vi "hidSPD Read Signal Board.vi"(8 "error in (no error)":errorcluster, 11 "spdDevSession in":T2={"spdRef"=0, "connected"=FALSE, "spdName"="", "specification"={"diod case"=enum."default", "type"=enum."Unknown", "frequency"=enum."Unknown"}, "hidSPD.Controller"={"TSet"=0.0, "HV_bias"=0.0, "DDS_stb_code"=0}, "hidSPD.Sturtup Values"={"TSet"=0.0, "HV_bias"=0.0, "DDS_stb_code"=0}} {"hidSPD.Sturtup Values"."HV_bias" format="%#_6p, V"; "hidSPD.Sturtup Values"."TSet" format="%#_6p, DegC"; "hidSPD.Controller"."HV_bias" format="%#_6p, V"; "hidSPD.Controller"."TSet" format="%#_6p, DegC"}) -> (0 "error out":errorcluster, 2 "Signal Board params":T1, 3 "spdDevSession out":T2={"spdRef"=0, "connected"=FALSE, "spdName"="", "specification"={"diod case"=enum."default", "type"=enum."Unknown", "frequency"=enum."Unknown"}, "hidSPD.Controller"={"TSet"=0.0, "HV_bias"=0.0, "DDS_stb_code"=0}, "hidSPD.Sturtup Values"={"TSet"=0.0, "HV_bias"=0.0, "DDS_stb_code"=0}} {"hidSPD.Sturtup Values"."HV_bias" format="%#_6p, V"; "hidSPD.Sturtup Values"."TSet" format="%#_6p, DegC"; "hidSPD.Controller"."HV_bias" format="%#_6p, V"; "hidSPD.Controller"."TSet" format="%#_6p, DegC"})   [LabVIEW 2018, in "hidSPDLibForLabView.lvlib"]
uses:
  hidSPDLibForLabView.lvlib
  hidSPD Controls/hidSPD Device Session.ctl
  hidSPD Controls/hidSPD.SPD specification.ctl
  hidSPD Controls/hidSPD SPD Diod Case.ctl
  hidSPD Controls/hidSPD SPD Type.ctl
  hidSPD Controls/hidSPD.STB Frequency.ctl
  hidSPD Controls/hidSPD Controller.ctl
  hidSPD Controls/hidSPD Controller Signal Report.ctl
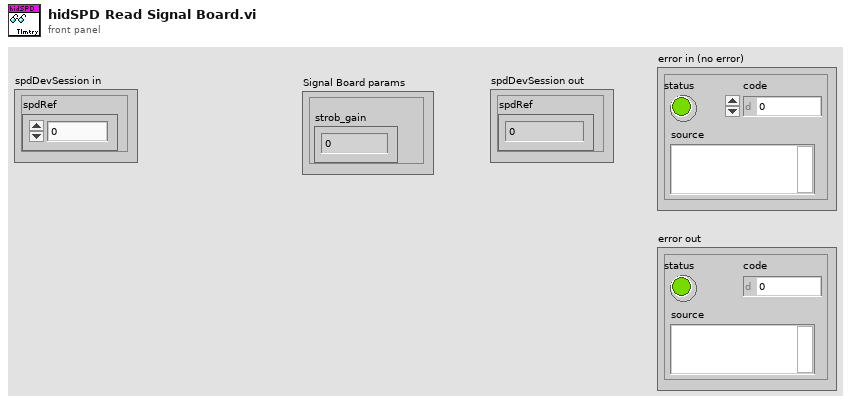
[diagram p1: front panel]
types:
  T1 = typedef "hidSPDLibForLabView.lvlib/hidSPD Controller Signal Report.ctl" = cluster{"strob_gain":i8, "receive_gain":i8, "positive_bias":i32, "negative_bias":i32, "deadtime":i16, "insensitivity":i16, "deadtime_strobe":i8, "dt_on":i8, "frequency":i16, "pllpwr":i8, "rvset":i16, "dvset":i16}
  T2 = typedef "hidSPDLibForLabView.lvlib/hidSPD Device Session.ctl" = cluster{"spdRef":u64, "connected":bool, "spdName":string, "specification":T3, "hidSPD.Controller":T7, "hidSPD.Sturtup Values":T7}
  T3 = typedef "hidSPDLibForLabView.lvlib/hidSPD.SPD specification.ctl" = cluster{"diod case":T4, "type":T5, "frequency":T6}
  T4 = typedef "hidSPDLibForLabView.lvlib/hidSPD SPD Diod Case.ctl" = enum16{"Unknown", "default", "butterfly"}
  T5 = typedef "hidSPDLibForLabView.lvlib/hidSPD SPD Type.ctl" = enum16{"Unknown", "Free Run", "Gate"}
  T6 = typedef "hidSPDLibForLabView.lvlib/hidSPD.STB Frequency.ctl" = enum16{"Unknown", "312", "1250"}
  T7 = typedef "hidSPDLibForLabView.lvlib/hidSPD Controller.ctl" = cluster{"TSet":sgl, "HV_bias":sgl, "DDS_stb_code":u16}
  T8 = enum16{"big-endian, network order", "native, host order", "little-endian"}
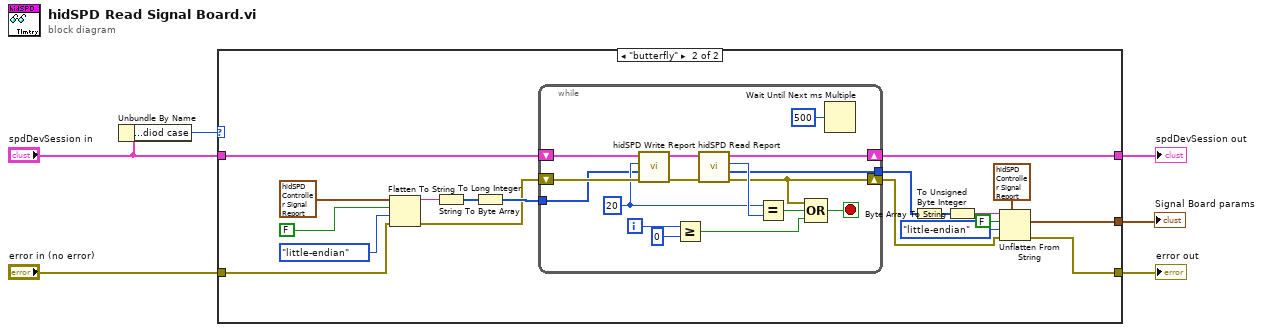
[diagram p0: block diagram]
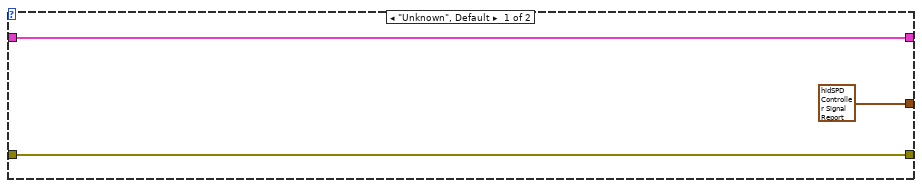
[diagram p2: hidden frame]
diagram:
  n1 = Unbundle By Name("spdDevSession in") -> ("specification.diod case"=w6:T4)
  n2 = case shown="\"butterfly\"" w6 {
    tunnel: "spdDevSession in" -> [w9 w28]
    tunnel: [w9 w27] -> w2
    tunnel: "error in (no error)" -> [w8 w19]
    tunnel: [w8 w11] -> w3
    tunnel: [T1 {"strob_gain"=-1, "receive_gain"=-1, "positive_bias"=-1, "negative_bias"=-1, "deadtime"=-1, "insensitivity"=-1, "deadtime_strobe"=-1, "dt_on"=-1, "frequency"=-1, "pllpwr"=-1, "rvset"=-1, "dvset"=-1} ("hidSPD Signal Setup Report") w10] -> w1
    frame "Unknown", Default {
    }
    frame "butterfly" {
      n3 = Flatten To String(anything=T1 {"strob_gain"=-1, "receive_gain"=-1, "positive_bias"=-1, "negative_bias"=-1, "deadtime"=-1, "insensitivity"=-1, "deadtime_strobe"=-1, "dt_on"=-1, "frequency"=-1, "pllpwr"=-1, "rvset"=-1, "dvset"=-1} ("hidSPD Signal Setup Report"), prepend array or string size? (T)=FALSE, byte order (0:big-endian, network order)=T8."little-endian", error in (no error)=w19) -> (data string=w26:string, error out=w20:errorcluster)  [unwired: 1 out]
      n4 = String To Byte Array(string=w26) -> (unsigned byte array=w25:u8[])
      n5 = To Long Integer(number=w25) -> (32bit integer=w21:i32[])
      n6 = while {
        shift-right: [w44] -> w27
        shift-left: w28 -> [w38]
        shift-right: [w40] -> w14
        shift-left: w20 -> [w37]
        tunnel: w21 -> [w30]
        tunnel: [w29] -> w13
        i -> [w33]
        stop <- w39 stop-if-true
        w36 = 20 ("cmd")
        n7 = call "hidSPD Write Report.vi"("error in (no error)"=w37, "data"=w30, "cmd"=w36, "spdDevSession in"=w38) -> ("error out"=w35:errorcluster, "spdDevSession out"=w34:T2)  [unwired: 6 in]
        n8 = Greater Or Equal?(x=w33, y=0) -> (x >= y?=w31:bool)
        n9 = call "hidSPD Read Report.vi"("error in (no error)"=w35, "spdDevSession in"=w34) -> ("error out"=w40:errorcluster, "data"=w29:i32[], "cmd"=w42:i32, "spdDevSession out"=w44:T2)  [unwired: 6 in]
        n10 = Equal?(x=w36, y=w42) -> (x = y?=w41:bool)
        n11 = Compound Arithmetic op=OR(w40, w41, w31) -> (w39:bool)
        n12 = Wait Until Next ms Multiple(millisecond multiple=u32 500) -> ()  [unwired: 1 out]
      }
      n13 = To Unsigned Byte Integer(number=w13) -> (unsigned 8bit integer=w12:u8[])
      n14 = Byte Array To String(unsigned byte array=w12) -> (string=w18:string)
      n15 = Unflatten From String(type=T1 {"strob_gain"=-1, "receive_gain"=-1, "positive_bias"=-1, "negative_bias"=-1, "deadtime"=-1, "insensitivity"=-1, "deadtime_strobe"=-1, "dt_on"=-1, "frequency"=-1, "pllpwr"=-1, "rvset"=-1, "dvset"=-1} ("hidSPD Signal Setup Report"), binary string=w18, data includes array or string size? (T)=FALSE, byte order (0:big-endian, network order)=T8."little-endian", error in (no error)=w14) -> (value=w10:T1, error out=w11:errorcluster)  [unwired: 1 out]
    }
  }
  "error out" <- w3
  "spdDevSession out" <- w2
  "Signal Board params" <- w1
